vi "UnoLoopbackTesterv2.vi"() -> ()   [LabVIEW 2009]
uses:
  <vilib>/Instr/_visa.llb/VISA Configure Serial Port (Instr).vi
panel:
  in  "stop":bool
  in  "System":enum32{"Main", "Serial Terminal"}(tab)=enum."Serial Terminal"
  out "Outgoing Messages":string
  in  "Send":bool
  out "Input":string
  in  "stop bits (10: 1 bit)":u16(ring)=10 items=["1.0"=10, "1.5"=15, "2.0"=20]
  in  "baud rate (9600)":u32=9600
  in  "parity (0:none)":enum16{"None", "Odd", "Even", "Mark", "Space"}(ring)
  in  "data bits (8)":u16=8 min=5 max=8 step=1
  in  "VISA resource name":refnum<visa-resource-name>
  out "Incoming Messages":string
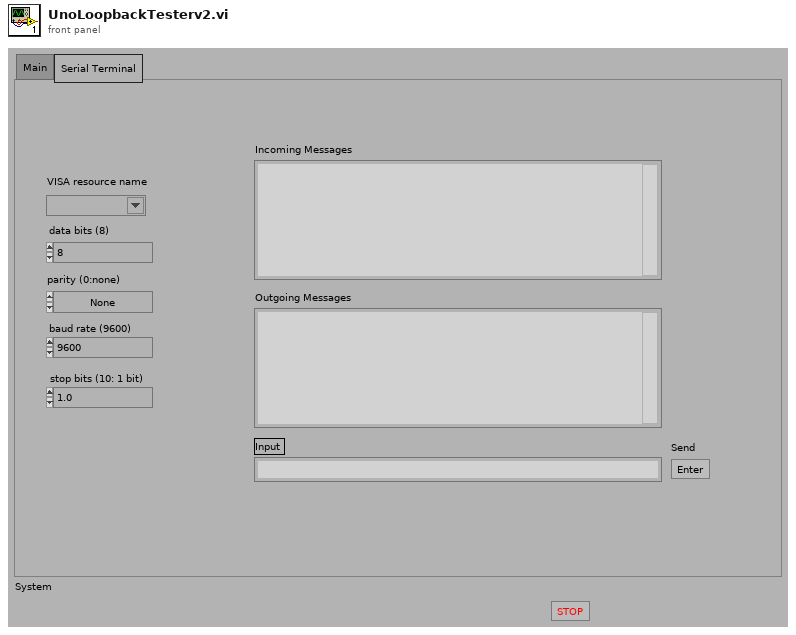
[diagram p1: front panel]
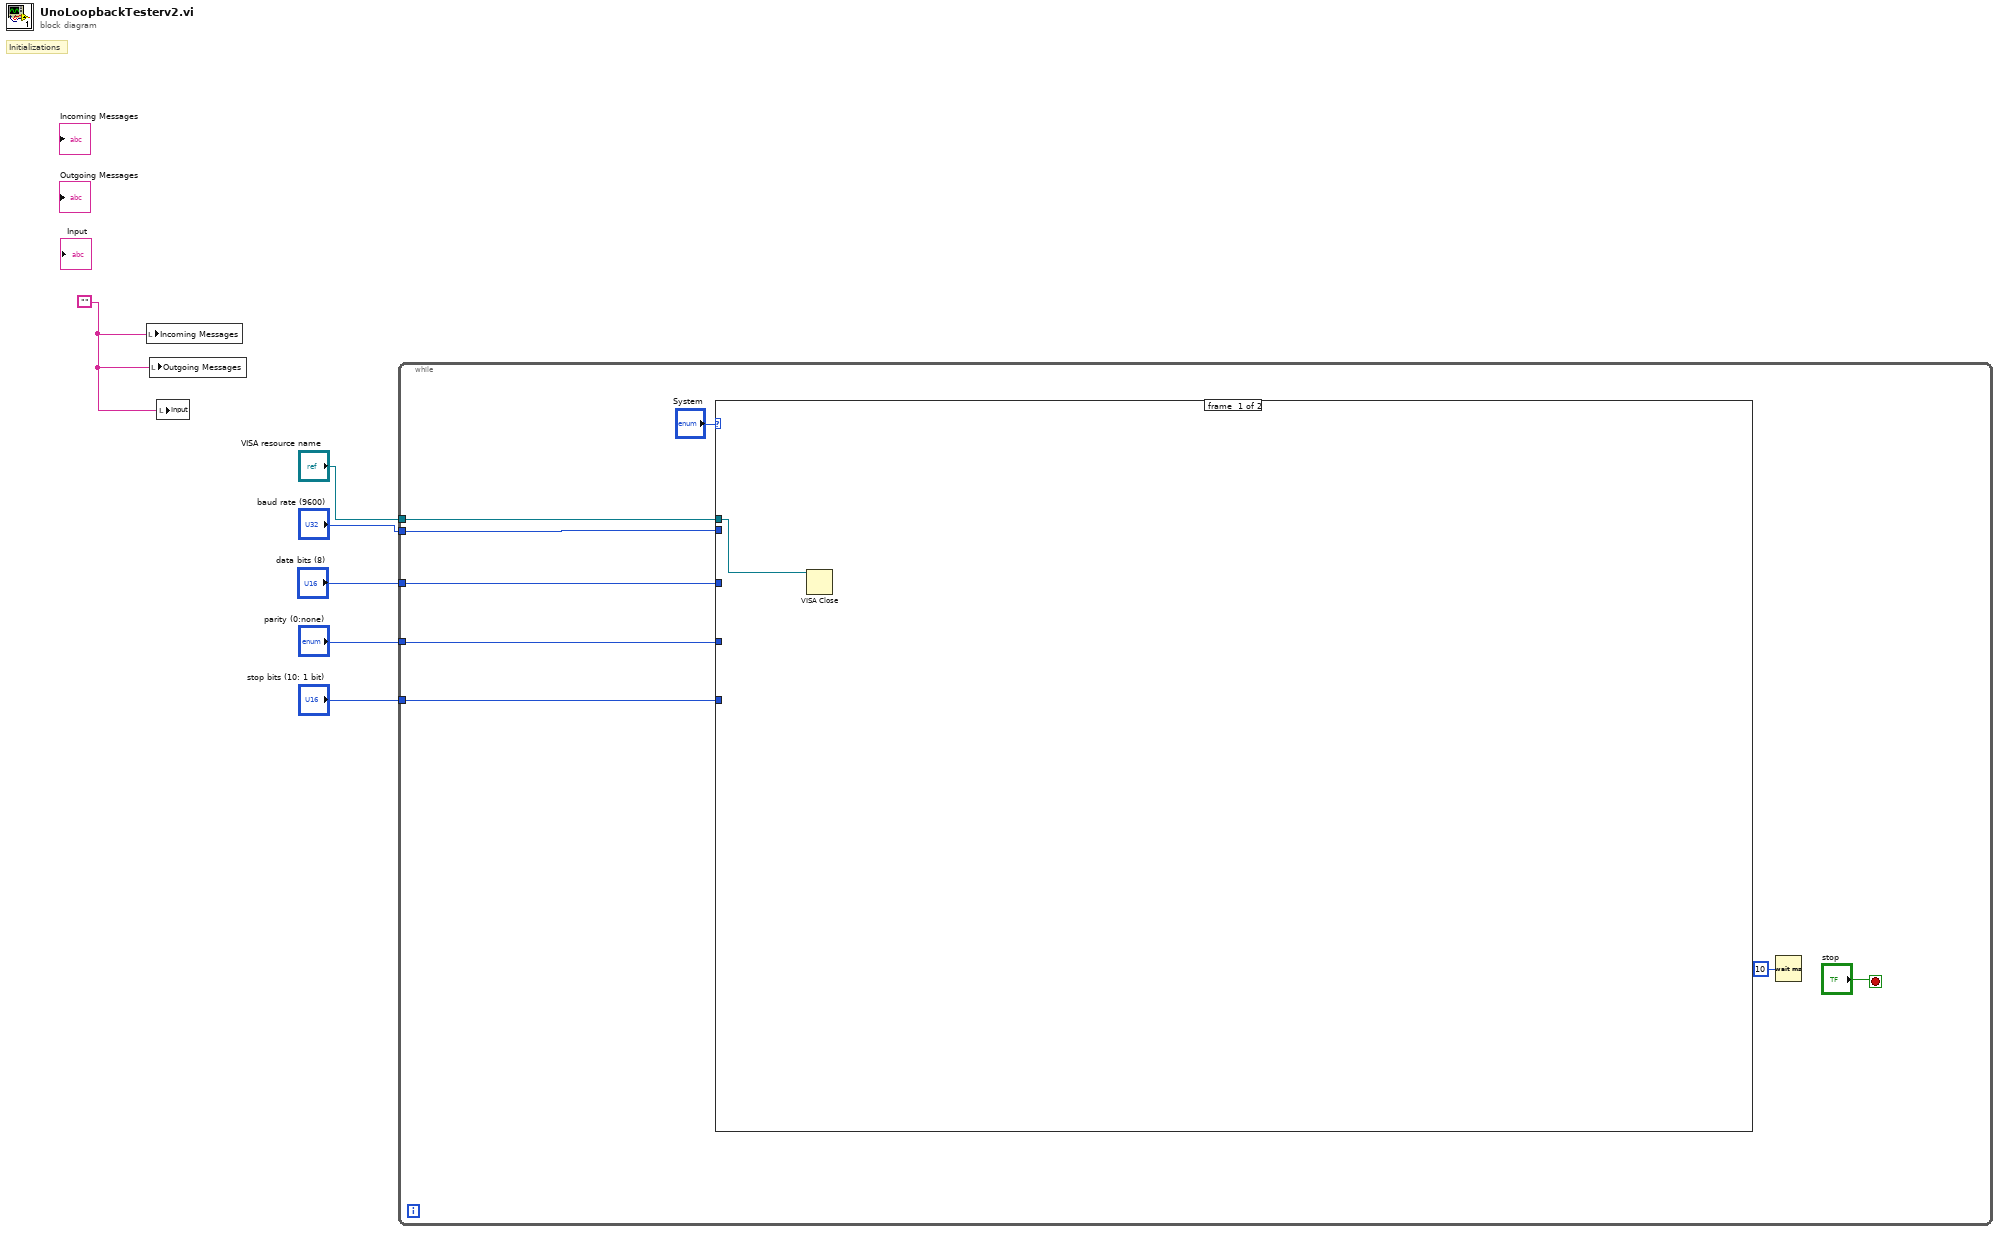
[diagram p0: block diagram]
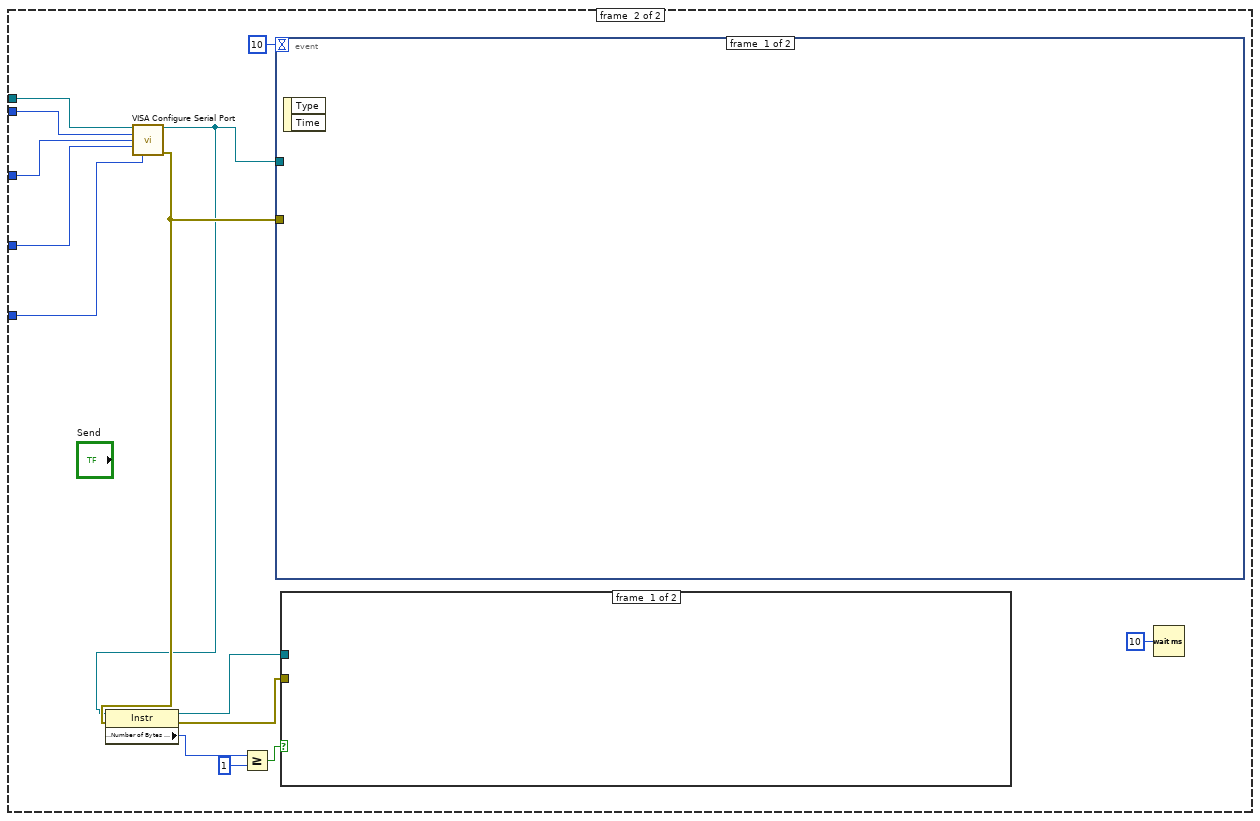
[diagram p2: hidden frame]
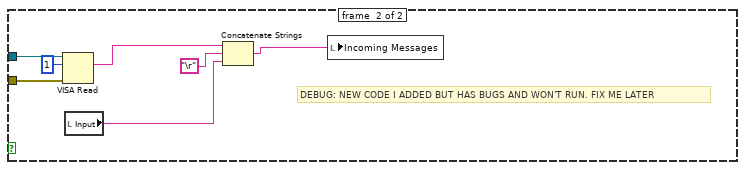
[diagram p3: hidden frame]
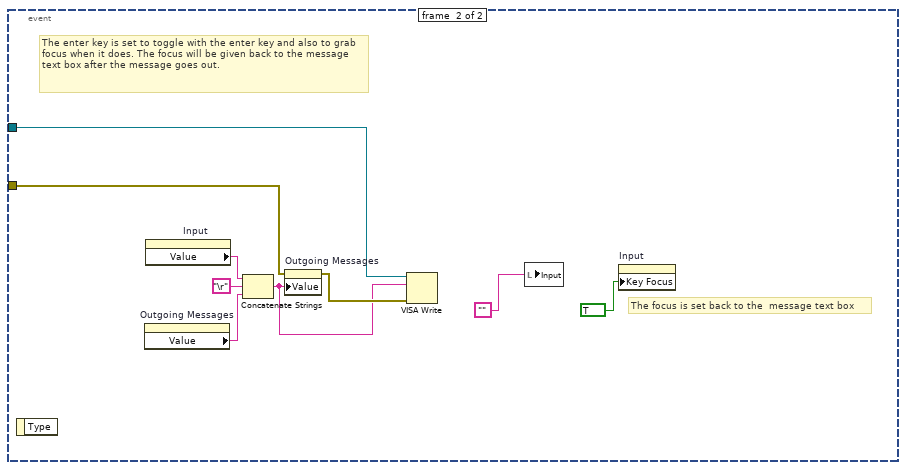
[diagram p4: hidden frame]
diagram:
  w1 = ""
  # "Initializations"
  n1 = local write "Incoming Messages"(w1) -> ()
  n2 = local write "Outgoing Messages"(w1) -> ()
  n3 = local write "Input"(w1) -> ()
  n4 = while {
    tunnel: "VISA resource name" -> [w11]
    tunnel: "baud rate (9600)" -> [w10]
    tunnel: "data bits (8)" -> [w9]
    tunnel: "parity (0:none)" -> [w8]
    tunnel: "stop bits (10: 1 bit)" -> [w7]
    stop <- "stop" stop-if-true
    n5 = case shown="\"Serial Terminal\"" "System" {
      tunnel: w11 -> [w15 w27]
      tunnel: w10 -> [_ w29]
      tunnel: w9 -> [_ w28]
      tunnel: w8 -> [_ w26]
      tunnel: w7 -> [_ w25]
      frame #0 {
        n6 = VISA Close(VISA resource name=w15) -> ()  [unwired: 1 in, 1 out]
      }
      frame #1 {
        n7 = call-poly "VISA Configure Serial Port"("VISA resource name"=w27, "baud rate (9600)"=w29, "data bits (8)"=w28, "parity (0:none)"=w26, "stop bits (10: 1 bit)"=w25) -> ("VISA resource name out"=w18:refnum<visa-resource-name>, "error out"=w19:errorcluster)  [unwired: 9 in]
        n8 = property class="Instr"(reference=w18, error in=w19) -> (reference out=w17:refnum<visa-resource-name>, error out=w16:errorcluster, "Serial Settings:Number of Bytes at Serial Port"=w22:u32)
        n9 = Greater Or Equal?(x=w22, y=u32 1) -> (x >= y?=w20:bool)
        n10 = event shown="[1] \"Send\": Value Change" {
          selector: _ -> [_ _]
          dyn-events: _ -> [_ _]
          timeout: 10 -> [_ _]
          tunnel: w18 -> [_ w39]
          tunnel: w19 -> [_ w38]
          event #0 {
            n11 = event-data() -> ()  [unwired: 1 in, 2 out]
          }
          event #1 {
            # "The enter key is set to toggle with the enter key and also to grab focus when it does. The focus will be given back to the message text box after the message goes out."
            # "The focus is set back to the  message text box"
            n12 = event-data() -> ()  [unwired: 1 in, 1 out]
            n13 = property on="Outgoing Messages" class="Str"() -> ("Value"=w43:string)  [unwired: 2 in, 2 out]
            n14 = property on="Input" class="Str"() -> ("Value"=w45:string)  [unwired: 2 in, 2 out]
            n15 = Concatenate Strings(w45, "\r", w43) -> (w40:string)
            n16 = property on="Outgoing Messages" class="Str"(error in=w38, "Value"=w40) -> (error out=w41:errorcluster)  [unwired: 1 in, 1 out]
            n17 = VISA Write(VISA resource name=w39, write buffer=w40, error in (no error)=w41) -> ()  [unwired: 3 out]
            n18 = local write "Input"("") -> ()
            n19 = property on="Input" class="Str"("Key Focus"=TRUE) -> ()  [unwired: 2 in, 2 out]
          }
        }
        n20 = case shown="True" w20 {
          tunnel: w17 -> [_ w36]
          tunnel: w16 -> [_ w35]
          frame #0 {
          }
          frame #1 {
            # "DEBUG: NEW CODE I ADDED BUT HAS BUGS AND WON'T RUN. FIX ME LATER"
            n21 = VISA Read(VISA resource name=w36, byte count=u32 1, error in (no error)=w35) -> (read buffer=w33:string)  [unwired: 3 out]
            n22 = local read "Input"() -> (w30:string)
            n23 = Concatenate Strings(w33, "\r", w30) -> (w31:string)
            n24 = local write "Incoming Messages"(w31) -> ()
          }
        }
        n25 = Wait (ms)(milliseconds to wait=u32 10) -> ()  [unwired: 1 out]
      }
    }
    n26 = Wait (ms)(milliseconds to wait=u32 10) -> ()  [unwired: 1 out]
  }
